vi "MecaDriveKinematics_Example.vi"() -> ()   [LabVIEW 2019]
uses:
  <vilib>/Rock Robotics/WPI/ThirdParty/JAS_Junk/TrajLib/TypeDef/CHASSIS_SPEEDS.ctl
  <vilib>/Rock Robotics/WPI/ThirdParty/JAS_Junk/TrajLib/Trajectory_Library.lvlib
panel:
  out "Rear Right\nVelocity Ft/Sec":dbl format="%13.2f"
  out "Rear Left\nVelocity Ft/Sec":dbl format="%13.2f"
  in  "Rear Right \nWheel Velocity\nFt/Sec":dbl
  in  "Rear Left \nWheel Velocity\nFT/Sec":dbl
  out "Front Right\nVelocity Ft/Sec":dbl format="%13.2f"
  out "Front Left\nVelocity Ft/Sec":dbl format="%13.2f"
  out "CHASSIS Speed\nM/S":T1 {"vOmega" format="%10.3f"; "vY" format="%10.3f"; "vX" format="%10.3f"}
  in  "Step":bool
  in  "Front Right \nWheel Velocity\nFt/Sec":dbl
  in  "Front Left \nWheel Velocity\nFT/Sec":dbl
  # "Mecanum Drive Kinematics Example"
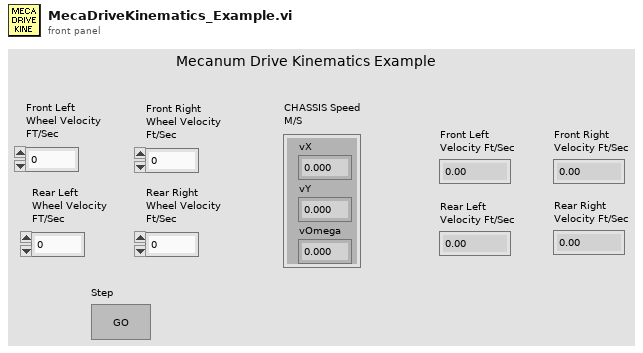
[diagram p1: front panel]
types:
  T1 = typedef "Trajectory_Library.lvlib/CHASSIS_SPEEDS.ctl" = cluster{"vX":dbl, "vY":dbl, "vOmega":dbl}
  T2 = typedef "Trajectory_Library.lvlib/TRANSLATION2D.ctl" = cluster{"X":dbl, "Y":dbl}
  T3 = typedef "Trajectory_Library.lvlib/MECA_DRIVE_KINEMATICS.ctl" = cluster{"FrontLeft":T2, "FrontRight":T2, "RearLeft":T2, "RearRight":T2, "InverseKinematics":T4, "ForwardKinematics":T4, "PrevCoR":T2}
  T4 = typedef "NI_Matrix.lvlib/RealMatrix.ctl" = dbl[][]
  T5 = typedef "Trajectory_Library.lvlib/MECA_WHEEL_SPEEDS.ctl" = cluster{"FrontLeftSpeed":dbl, "FrontRightSpeed":dbl, "RearLeftSpeed":dbl, "RearRightSpeed":dbl}
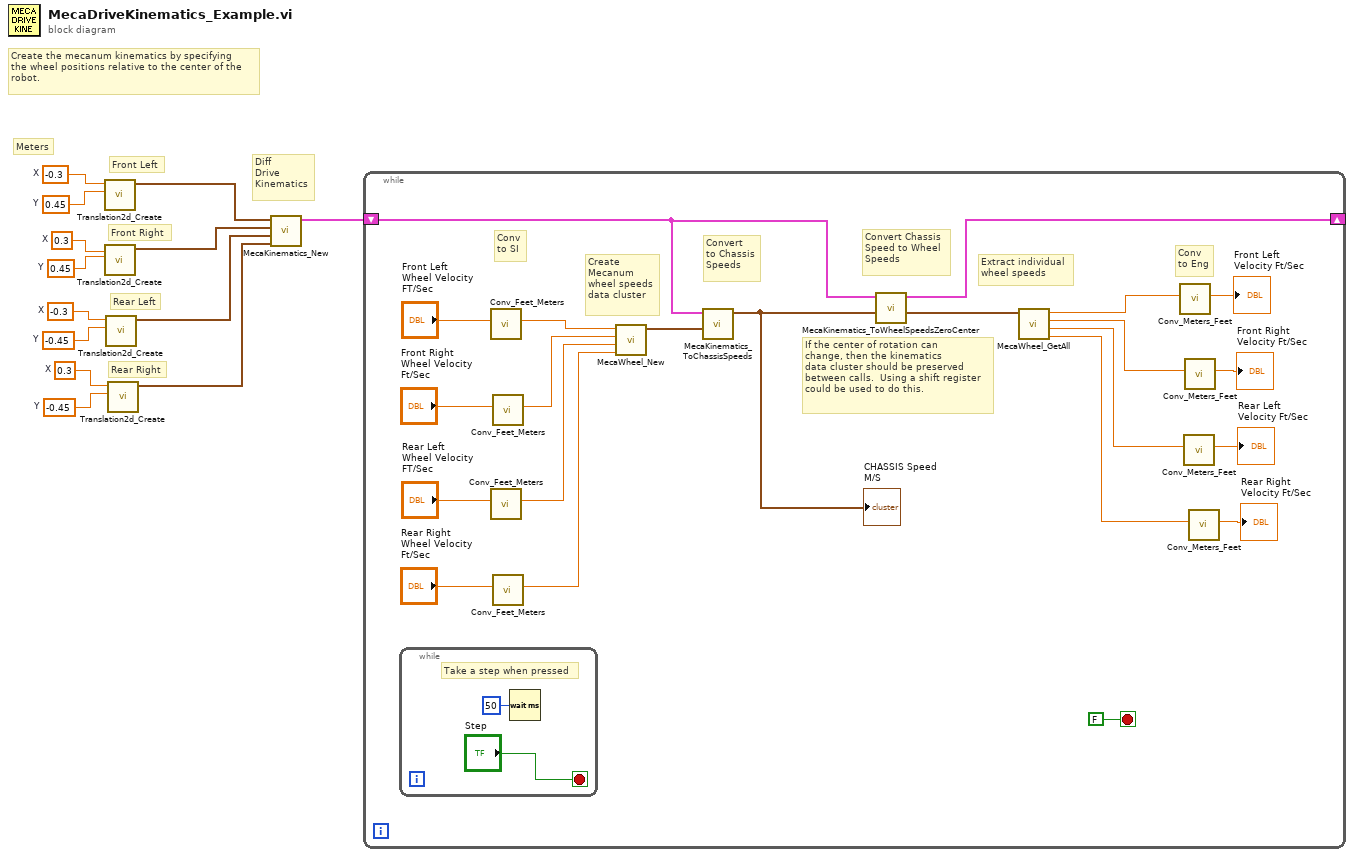
[diagram p0: block diagram]
diagram:
  w6 = -0.3  # X
  w7 = 0.45  # Y
  w8 = 0.3  # X
  w9 = 0.45  # Y
  w10 = -0.3  # X
  w11 = -0.45  # Y
  w12 = 0.3  # X
  w13 = -0.45  # Y
  # "Meters"
  # "Rear Right"
  # "Rear Left"
  # "Front Right"
  # "Front Left"
  # "Create the mecanum kinematics by specifying\nthe wheel positions relative to the center of the\nrobot."
  # "Diff\nDrive\nKinematics"
  n1 = call <vilib>:"Translation2d_Create.vi"("Y"=w7, "X"=w6) -> ("TRANSLATION"=w5:T2)  [unwired: 9 in]
  n2 = call <vilib>:"Translation2d_Create.vi"("Y"=w9, "X"=w8) -> ("TRANSLATION"=w4:T2)  [unwired: 9 in]
  n3 = call <vilib>:"Translation2d_Create.vi"("Y"=w11, "X"=w10) -> ("TRANSLATION"=w3:T2)  [unwired: 9 in]
  n4 = call <vilib>:"Translation2d_Create.vi"("Y"=w13, "X"=w12) -> ("TRANSLATION"=w2:T2)  [unwired: 9 in]
  n5 = call <vilib>:"MecaKinematics_New.vi"("RearRight"=w2, "RearLeft"=w3, "FrontRight"=w4, "FrontLeft"=w5) -> ("MECA_DRIVE_KINEMATICS"=w1:T3)  [unwired: 7 in]
  n6 = while {
    shift-right: [w19] -> _
    shift-left: w1 -> [w18]
    stop <- FALSE stop-if-true
    # "If the center of rotation can\nchange, then the kinematics\ndata cluster should be preserved\nbetween calls.  Using a shift register\ncould be used to do this."
    # "Extract individual\nwheel speeds"
    # "Conv\nto Eng"
    # "Create\nMecanum\nwheel speeds\ndata cluster"
    # "Conv\nto SI"
    # "Convert Chassis\nSpeed to Wheel\nSpeeds"
    # "Convert\nto Chassis\nSpeeds"
    n7 = while {
      stop <- "Step" stop-if-true
      # "Take a step when pressed"
      n8 = Wait (ms)(milliseconds to wait=u32 50) -> ()  [unwired: 1 out]
    }
    n9 = call <vilib>:"Conv_Feet_Meters.vi"("Feet"="Front Left \nWheel Velocity\nFT/Sec") -> ("Meters"=w26:dbl)  [unwired: 10 in]
    n10 = call <vilib>:"Conv_Feet_Meters.vi"("Feet"="Rear Left \nWheel Velocity\nFT/Sec") -> ("Meters"=w24:dbl)  [unwired: 10 in]
    n11 = call <vilib>:"Conv_Feet_Meters.vi"("Feet"="Front Right \nWheel Velocity\nFt/Sec") -> ("Meters"=w25:dbl)  [unwired: 10 in]
    n12 = call <vilib>:"Conv_Feet_Meters.vi"("Feet"="Rear Right \nWheel Velocity\nFt/Sec") -> ("Meters"=w23:dbl)  [unwired: 10 in]
    n13 = call <vilib>:"MecaWheel_New.vi"("RearRightSpeed"=w23, "RearLeftSpeed"=w24, "FrontRightSpeed"=w25, "FrontLeftSpeed"=w26) -> ("MECA_WHEEL_SPEEDS"=w29:T5)  [unwired: 7 in]
    n14 = call <vilib>:"MecaKinematics_ToChassisSpeeds.vi"("MECA_WHEEL_SPEEDS"=w29, "in MECA_DRIVE_KINEMATICS"=w18) -> ("ChassisSpeeds"=w33:T1)  [unwired: 9 in]
    "CHASSIS Speed\nM/S" <- w33
    n15 = call <vilib>:"MecaKinematics_ToWheelSpeedsZeroCenter.vi"("ChassisSpeeds"=w33, "in MECA_DRIVE_KINEMATICS"=w18) -> ("MECA_WHEEL_SPEEDS"=w20:T5, "out MECA_DRIVE_KINEMATICS"=w19:T3)  [unwired: 8 in]
    n16 = call <vilib>:"MecaWheel_GetAll.vi"("MECA_WHEEL_SPEEDS"=w20) -> ("RearRightSpeed"=w14:dbl, "RearLeftSpeed"=w15:dbl, "FrontRightSpeed"=w16:dbl, "FrontLeftSpeed"=w17:dbl)  [unwired: 7 in]
    n17 = call <vilib>:"Conv_Meters_Feet.vi"("Meters"=w17) -> ("Feet"=→"Front Left\nVelocity Ft/Sec":dbl)  [unwired: 10 in]
    n18 = call <vilib>:"Conv_Meters_Feet.vi"("Meters"=w15) -> ("Feet"=→"Rear Left\nVelocity Ft/Sec":dbl)  [unwired: 10 in]
    n19 = call <vilib>:"Conv_Meters_Feet.vi"("Meters"=w16) -> ("Feet"=→"Front Right\nVelocity Ft/Sec":dbl)  [unwired: 10 in]
    n20 = call <vilib>:"Conv_Meters_Feet.vi"("Meters"=w14) -> ("Feet"=→"Rear Right\nVelocity Ft/Sec":dbl)  [unwired: 10 in]
  }
